vi "Initialize.vi"(8 "error in (no error)":errorcluster, 11 "Ballard ARINC-429 Tx Execution Unit in":refnum<class "Ballard ARINC-429 Tx Execution Unit.lvclass">) -> (0 "error out":errorcluster, 3 "Ballard ARINC-429 Tx Execution Unit out":refnum<class "Ballard ARINC-429 Tx Execution Unit.lvclass">)   [LabVIEW 2020, in "Communication Bus Template Engine.lvlib" / "Implementation.lvlib" / "Ballard ARINC-429 Tx Execution Unit.lvclass"]
uses:
  Ballard ARINC-429 Tx Execution Unit.lvclass
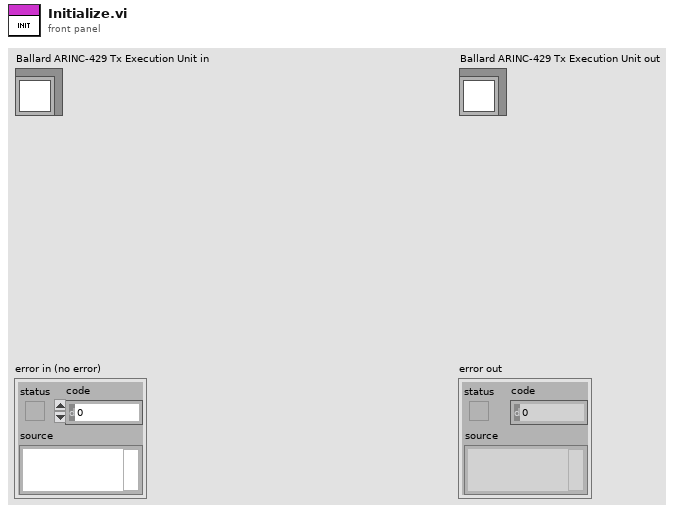
[diagram p1: front panel]
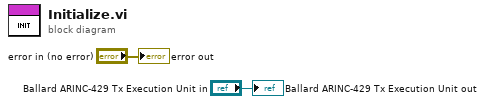
[diagram p0: block diagram]
diagram:
  "error out" <- "error in (no error)"
  "Ballard ARINC-429 Tx Execution Unit out" <- "Ballard ARINC-429 Tx Execution Unit in"
